vi "Actor Core.vi"(8 "error in":errorcluster, 11 "AI_Task in":refnum<class "AI_Task.lvclass">) -> (0 "error out":errorcluster, 3 "Actor out":refnum<class "Actor.lvclass">)   [LabVIEW 2025, in "AI_Task.lvlib" / "AI_Task.lvclass"]
doc: "<p>(<strong>Filename</strong>: <span class=\"dnl\">Actor Framework.lvlib:Actor.lvclass:Actor Core.vi</span>)</p>\n<p>Receives messages to the actor, reacts to them, and initiates any error handling that may shut the actor down.</p>\n<p>Descendant classes may override this VI to append parallel tasks for the actor to complete while it handles messages. Overrides use the <a href=\"nihelplauncher://docs/csh?context=lvcore_glang_udclass\">Call Parent Class Method</a> node.</p>"
uses:
  AI_Task.lvclass
  <vilib>/ActorFramework/Actor/Actor.lvclass
  AI_Task.lvclass/AI_Task.ctl
  <vilib>/ActorFramework/Actor/Actor.lvclass/Actor.ctl
  <vilib>/ActorFramework/Message Enqueuer/Message Enqueuer.lvclass/Message Enqueuer.ctl
  AI_Task Messages/SwitchChart Msg/SwitchChart Msg.lvclass/SwitchChart Msg.ctl
  <vilib>/ActorFramework/Message Enqueuer/Init from Existing Queue.vi
  <vilib>/ActorFramework/Message Enqueuer/Enqueue.vi
  AI_Task Messages/SwitchChart Msg/SwitchChart Msg.lvclass
  <vilib>/ActorFramework/Message Priority Queue/Priority Enqueue.vi
  <vilib>/ActorFramework/Message Enqueuer/Message Enqueuer.lvclass
  Task_Abstr/Task_Abstr/Task_Abstr.lvclass
panel:
  out "Waveform Graph":waveform(dbl)[](graph)
  out "Waveform Chart":waveform(dbl)[](graph)
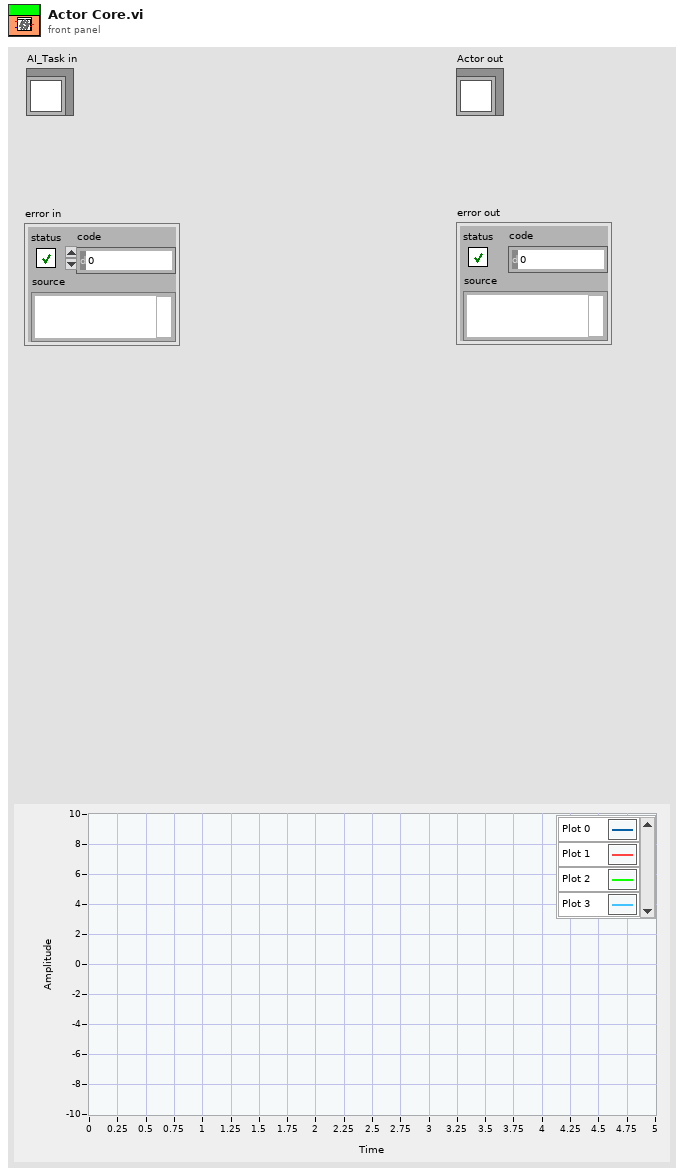
[diagram p1: front panel]
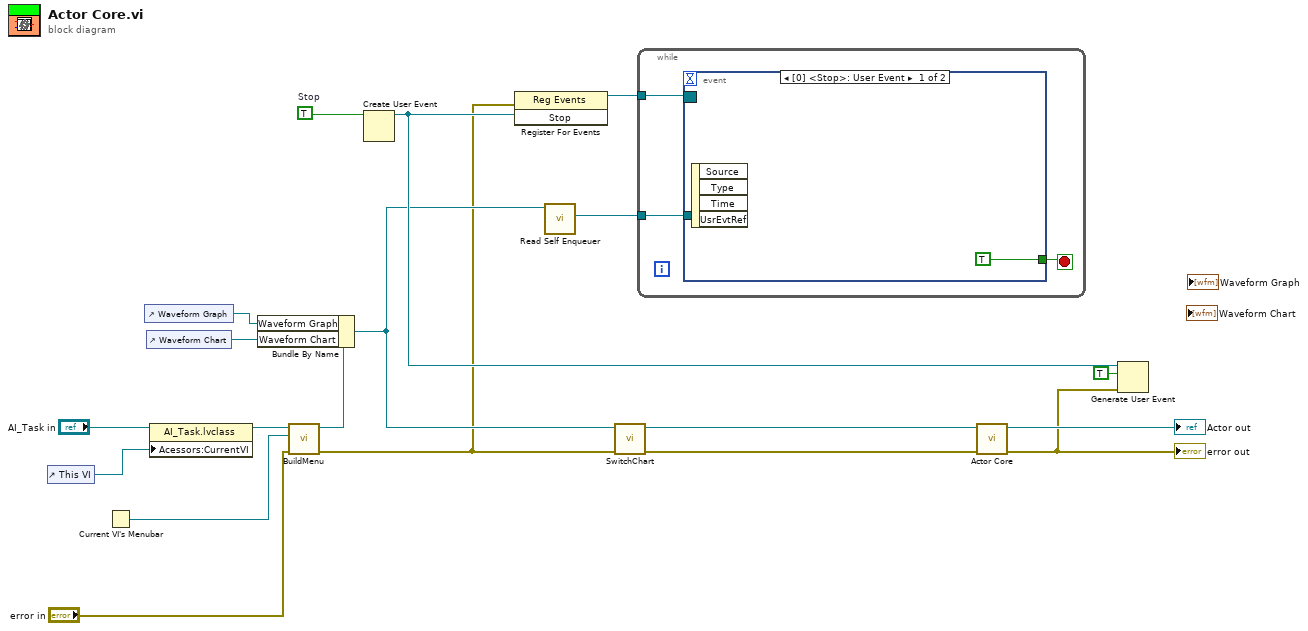
[diagram p0: block diagram]
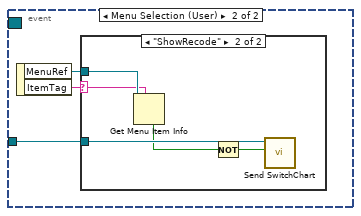
[diagram p2: hidden frame]
diagram:
  w15 = TRUE  # Stop
  n1 = control-ref of="This VI"() -> (w17:refnum<vi>)
  n2 = Current VI's Menubar() -> (w7:refnum<k9>)
  n3 = control-ref of="Waveform Graph"() -> (w6:refnum<vi>)
  n4 = control-ref of="Waveform Chart"() -> (w16:refnum<vi>)
  n5 = property class="AI_Task.lvclass"(reference="AI_Task in", "Acessors:CurrentVI"=w17) -> (reference out=w9:refnum<class "AI_Task.lvclass">)  [unwired: 1 in, 1 out]
  n6 = call "BuildMenu.vi"("error in (no error)"="error in", "menu reference"=w7, "AI_Task in"=w9) -> ("error out"=w2:errorcluster, "AI_Task out"=w8:refnum<class "AI_Task.lvclass">)  [unwired: 7 in]
  n7 = Bundle By Name(cluster=w8, "Waveform Graph"=w6, "Waveform Chart"=w16) -> (w5:refnum<class "AI_Task.lvclass">)
  n8 = Create User Event(user event datatype=w15) -> (user event=w12:refnum<user-event>)  [unwired: 1 in, 1 out]
  n9 = register-events(error in=w2, w12) -> (reference out=w14:refnum<event-registration>)  [unwired: 1 in, 1 out]
  n10 = call <vilib>:"Read Self Enqueuer.vi"("Actor"=w5) -> ("Self Enqueuer"=w10:refnum<class "Message Enqueuer.lvclass">)  [unwired: 10 in]
  n11 = call "SwitchChart.vi"("error in (no error)"=w2, "AI_Task in"=w5) -> ("error out"=w3:errorcluster, "AI_Task out"=w4:refnum<class "AI_Task.lvclass">)  [unwired: 8 in]
  n12 = while {
    tunnel: w14 -> [w22]
    tunnel: w10 -> [w20]
    stop <- w21 stop-if-true
    n13 = event shown="[0] <Stop>: User Event" {
      selector: w22 -> [_ _]
      dyn-events: _ -> [_ _]
      timeout: _ -> [_ _]
      tunnel: [TRUE _] -> w21
      tunnel: w20 -> [_ w25]
      event User Event {
        n14 = event-data() -> ()  [unwired: 1 in, 4 out]
      }
      event Menu Selection (User) {
        n15 = event-data() -> ("MenuRef"=w24:refnum<k9>, "ItemTag"=w26:string)  [unwired: 1 in]
        n16 = case shown="\"ShowRecode\"" w26 {
          selector: w26 -> [_ w29]
          tunnel: w25 -> [_ w31]
          tunnel: w24 -> [_ w30]
          frame Default {
          }
          frame "ShowRecode" {
            n17 = Get Menu Item Info(7:w29, 11:w30) -> (4:w28:bool)  [unwired: 1 in, 6 out]
            n18 = Not(x=w28) -> (.not. x?=w27:bool)
            n19 = call "Send SwitchChart.vi"("Switch"=w27, "Message Enqueuer"=w31) -> ()  [unwired: 8 in, 2 out]
          }
        }
      }
    }
  }
  n20 = call-parent "Actor Core.vi"("error in"=w3, "Task_Abstr in"=w4) -> ("error out"=w13:errorcluster, "Actor out"=→"Actor out":refnum<class "Actor.lvclass">)  [unwired: 8 in]
  "error out" <- w13
  n21 = Generate User Event(user event=w12, event data cluster=TRUE ("event data"), error in=w13) -> ()  [unwired: 1 in, 2 out]
